vi "Read Local Msg Set.vi"(11 "Actor in":refnum<class "Actor.lvclass">) -> (2 "Local Msg Set":T1)   [LabVIEW 2025, in "jettl.lvlib" / "Actor.lvclass"]
uses:
  Actor.lvclass
  Msg Set.ctl
  Msg/Msg.lvclass
  jettl.lvlib
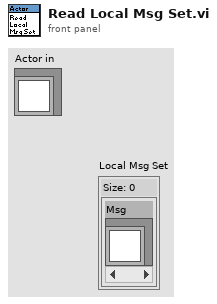
[diagram p1: front panel]
types:
  T1 = typedef "jettl.lvlib/Msg Set.ctl" = set{refnum<class "Msg.lvclass">}
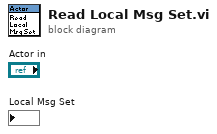
[diagram p0: block diagram]
diagram:
